vi "to string 3.2.vi"(8 "error in":errorcluster, 10 "data in":string, 11 "Shared Memory configuration in":refnum<class "Shared Memory configuration.lvclass">) -> (0 "error out":errorcluster, 2 "data out":string, 3 "Shared Memory configuration out":refnum<class "Shared Memory configuration.lvclass">)   [LabVIEW 2013, in "Shared Memory configuration.lvclass"]
uses:
  Shared Memory configuration.lvclass
  Shared Memory configuration.lvclass/Shared Memory configuration.ctl
  <vilib>/NI/Configuration Framework/serializable configuration/NISE_CEF_serializable configuration.lvclass
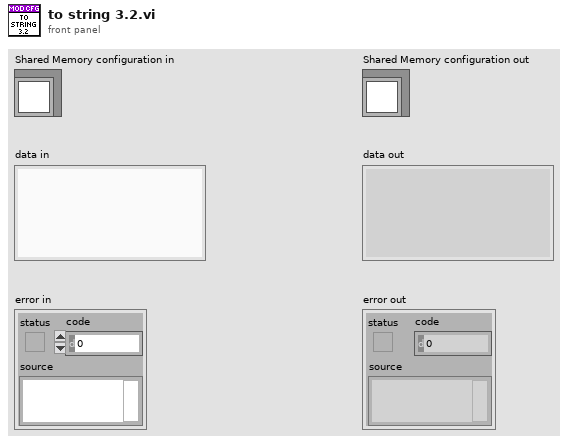
[diagram p1: front panel]
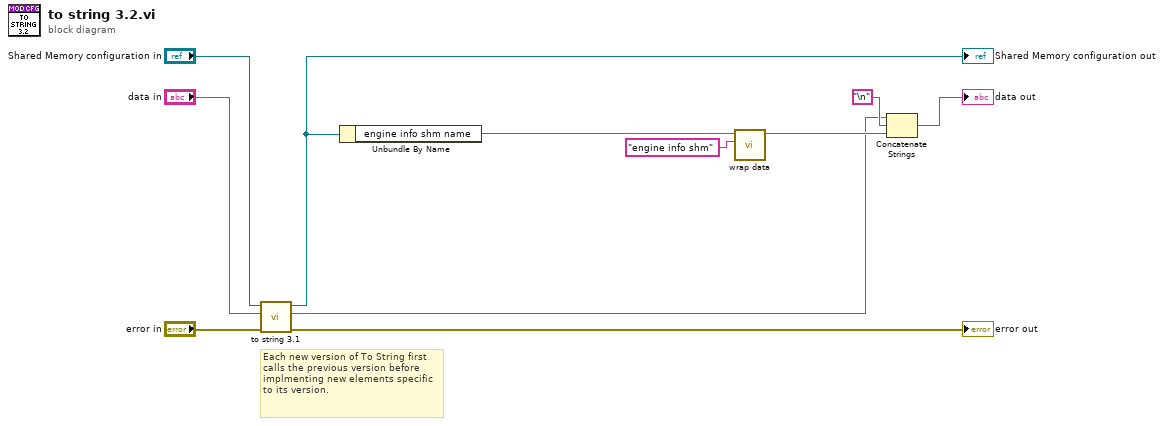
[diagram p0: block diagram]
diagram:
  # "Each new version of To String first calls the previous version before implmenting new elements specific to its version."
  n1 = call "to string 3.1.vi"("error in"="error in", "data in"="data in", "Shared Memory configuration in"="Shared Memory configuration in") -> ("error out"=→"error out":errorcluster, "data out"=w3:string, "Shared Memory configuration out"=w5:refnum<class "Shared Memory configuration.lvclass">)  [unwired: 6 in]
  "Shared Memory configuration out" <- w5
  n2 = Unbundle By Name(w5) -> ("engine info shm name"=w1:string)
  n3 = call <vilib>:"wrap data.vi"("identifier"="engine info shm", "data to wrap"=w1) -> ("wrapped data"=w8:string)  [unwired: 9 in]
  n4 = Concatenate Strings(w3, "\n", w8) -> (→"data out":string)
